vi "数组字符串解码-字符串至数组.vi"(0 "字符串":string, 1 "分隔字符串":string="#") -> (2 "数组":string[](array[string]))   [LabVIEW 2014]
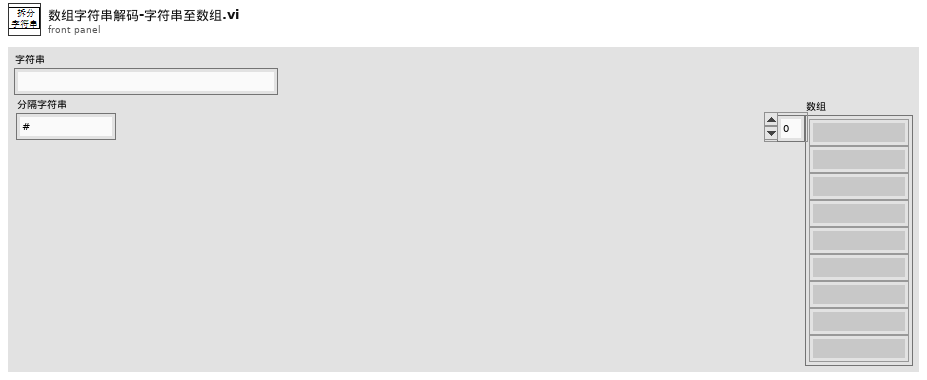
[diagram p1: front panel]
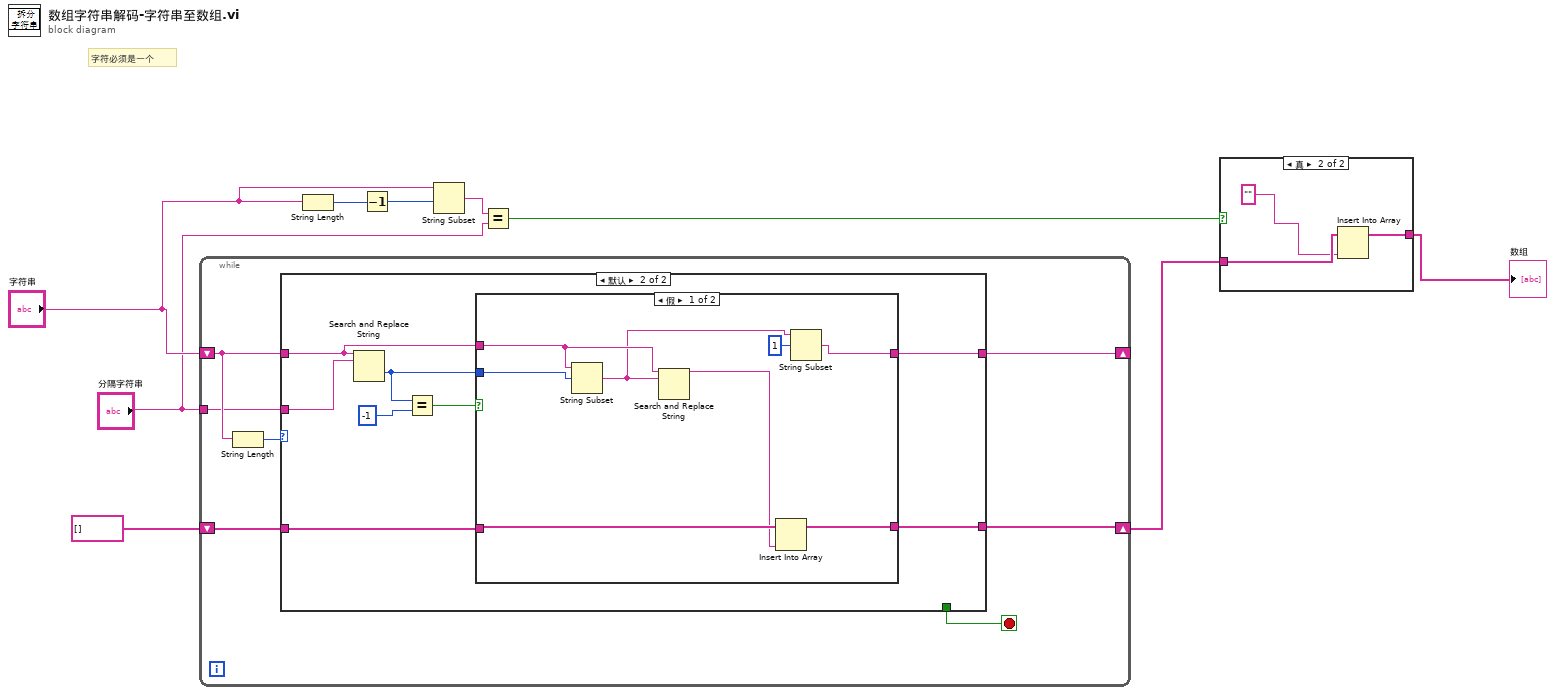
[diagram p0: block diagram]
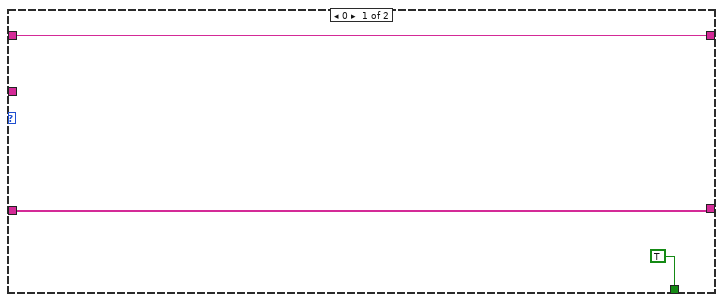
[diagram p3: hidden frame]
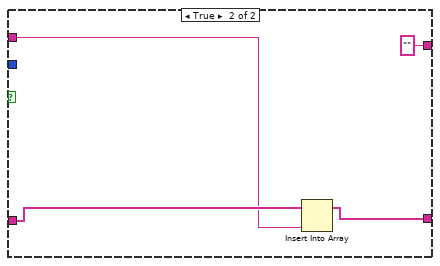
[diagram p4: hidden frame]
diagram:
  # "字符必须是一个"
  n1 = while {
    shift-right: [w15] -> w3
    shift-left: string[] [] -> [w16]
    shift-right: [w11] -> _
    shift-left: "字符串" -> [w13]
    tunnel: "分隔字符串" -> [w10]
    stop <- w12 stop-if-true
    n2 = String Length(string=w13) -> (length=w14:i32)
    n3 = case shown="默认" w14 {
      tunnel: w13 -> [w17 w25]
      tunnel: w16 -> [w19 w23]
      tunnel: [w19 w22] -> w15
      tunnel: [TRUE _] -> w12
      tunnel: [w17 w21] -> w11
      tunnel: w10 -> [_ w20]
      frame 0 {
      }
      frame Default {
        n4 = Search and Replace String(input string=w25, search string=w20) -> (offset past replacement=w24:i32)  [unwired: 6 in, 3 out]
        n5 = Equal?(x=w24, y=-1) -> (x = y?=w26:bool)
        n6 = case shown="假" w26 {
          tunnel: w25 -> [w31 w37]
          tunnel: w24 -> [w35 _]
          tunnel: w23 -> [w34 w38]
          tunnel: [w32 w36] -> w22
          tunnel: [w29 ""] -> w21
          frame False {
            n7 = String Subset(string=w31, offset (0)=w35) -> (substring=w28:string)  [unwired: 1 in]
            n8 = Search and Replace String(input string=w31, search string=w28) -> (result string=w33:string)  [unwired: 6 in, 3 out]
            n9 = Insert Into Array(array=w34, new element=w33) -> (w32:string[])  [unwired: 1 in]
            n10 = String Subset(string=w28, offset (0)=1 ("偏移量(0)")) -> (substring=w29:string)  [unwired: 1 in]
          }
          frame True {
            n11 = Insert Into Array(array=w38, new element=w37) -> (w36:string[])  [unwired: 1 in]
          }
        }
      }
    }
  }
  n12 = String Length(string="字符串") -> (length=w7:i32)
  n13 = Decrement(x=w7) -> (x-1=w1:i32)
  n14 = String Subset(string="字符串", offset (0)=w1) -> (substring=w6:string)  [unwired: 1 in]
  n15 = Equal?(x=w6, y="分隔字符串") -> (x = y?=w4:bool)
  n16 = case shown="真" w4 {
    tunnel: w3 -> [w40 w43]
    tunnel: [w40 w42] -> w2
    frame False {
    }
    frame True {
      n17 = Insert Into Array(array=w43, new element="" ("结果字符串")) -> (w42:string[])  [unwired: 1 in]
    }
  }
  "数组" <- w2
